vi "Goto Point Continously.vi"(10 "Stop Motors":bool, 11 "OH SHIT, STOP":bool) -> ()   [LabVIEW 2017]
uses:
  <vilib>/Platform/TimedLoop/XDataNode/wakeup.ctl
  <vilib>/Platform/TimedLoop/XDataNode/XDNodeRunTimeDep.lvlib
  <vilib>/Platform/TimedLoop/XDataNode/nitl_modes.ctl
  <vilib>/Platform/TimedLoop/XDataNode/timing_clust.ctl
  <vilib>/Platform/TimedLoop/XDataNode/XDataNode.xnode
  Globals/Pose.vi
  Globals/Target Pose.vi
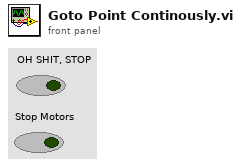
[diagram p1: front panel]
types:
  T1 = typedef "XDNodeRunTimeDep.lvlib/timing_clust.ctl" = cluster{"Expected End [f-1]":u64, "Actual End [f-1]":u64, "Finished Late? [f-1]":bool, "Expected End [i-1]":u64, "Actual End [i-1]":u64, "Finished Late? [i-1]":bool, "Expected Start [i]":u64, "Actual Start [i]":u64, "Expected Start [f]":u64, "Actual Start [f]":u64, "Source Name":string, "Structure Name":string, "Period":i64, "Deadline":i64, "Offset":i64, "Start":i64, "Priority":i32, "Timeout":i32, "Mode":T2, "Wakeup Reason":T3, "Error":errorcluster, "Source Type":string, "Secondary Source Type":string, "Global End Time":u64, "Global Start Time":u64, "Frame Duration":u64, "Iteration Duration":u64, "Assigned CPU":i32, "I/O Scan Engine Mode":u32}
  T2 = typedef "XDNodeRunTimeDep.lvlib/nitl_modes.ctl" = enum32{"No Change", "Process missed periods, maintain original phase", "Discard missed periods, maintain original phase", "Process missed periods, ignore original phase", "Discard missed periods, ignore original phase"}
  T3 = typedef "XDNodeRunTimeDep.lvlib/wakeup.ctl" = enum32{"Normal", "Aborted", "Asynchronous wakeup", "Timing source error", "Timed loop error", "Timeout"}
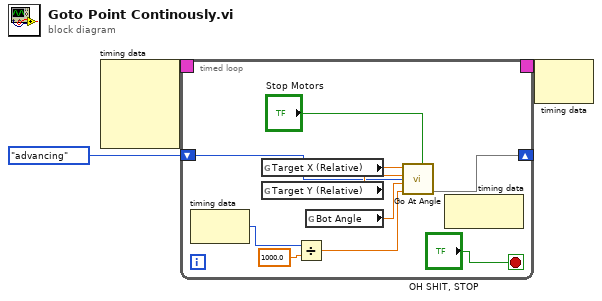
[diagram p0: block diagram]
diagram:
  n1 = node-c288() -> (w3:T1)  [unwired: 4 in]
  n2 = timed-loop {
    timing: w3 -> [_]
    timing-out: [_] -> w2
    shift-right: [w7] -> _
    shift-left: enum16{"turning", "advancing"}."advancing" ("New state") -> [w6]
    stop <- "OH SHIT, STOP" stop-if-true
    n3 = node-c288() -> (w12:i64)  [unwired: 1 in]
    n4 = global read "Target Pose.vi" "Target X (Relative)"() -> (w11:dbl)
    n5 = global read "Target Pose.vi" "Target Y (Relative)"() -> (w10:dbl)
    n6 = Divide(x=w12, y=1000.0) -> (x/y=w8:dbl)
    n7 = global read "Pose.vi" "Bot Angle"() -> (w9:dbl)
    n8 = call "Go At Angle.vi"("Target Angle"=w11, 1:w10, "Bot Angle"=w9, "dt"=w8, 4:w6, "Stop motors"="Stop Motors") -> (10:w7)  [unwired: 4 in]
    n9 = node-c288() -> ()  [unwired: 1 in, 1 out]
  }
  n10 = node-c288(w2) -> ()  [unwired: 1 out]
